vi "SUB_Verify_RandomCode.vi"() -> (1 "Boolean":bool=TRUE)   [LabVIEW 2011]
uses:
  <vilib>/event_ctls.llb/eventvkey.ctl
panel:
  in  "請鍵入如上的驗證碼":string="192.168.1.3\n192.168.1.1\n192.168.1.1"
  out "驗證碼":dbl format="%#_9g"
  # "KT300IP 測點 FAE 使用"
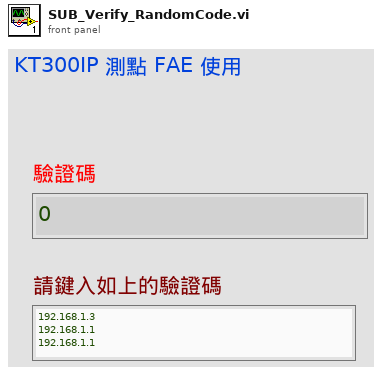
[diagram p1: front panel]
types:
  T1 = typedef "eventvkey.ctl" = enum16{"ASCII", "Enter", "Return", "Shift", "Ctrl", "Alt", "Cmd", "Opt", "Caps", "NumLock", "Clear", "Break", "Up", "Down", "Left", "Right", "Insert", "Delete", "Home", "End", "PageUp", "PageDown", "Escape", "Help", "Pause", "ScrollLock", "F1", "F2", "F3", "F4", "F5", "F6", "F7", "F8", "F9", "F10", "F11", "F12", "F13", "F14", "F15", "F16", "F17", "F18", "F19", "F20", "F21", "F22", "F23", "F24", "Play", "VolumeUp", "VolumeDown", "Mute", "Two Byte Char"}
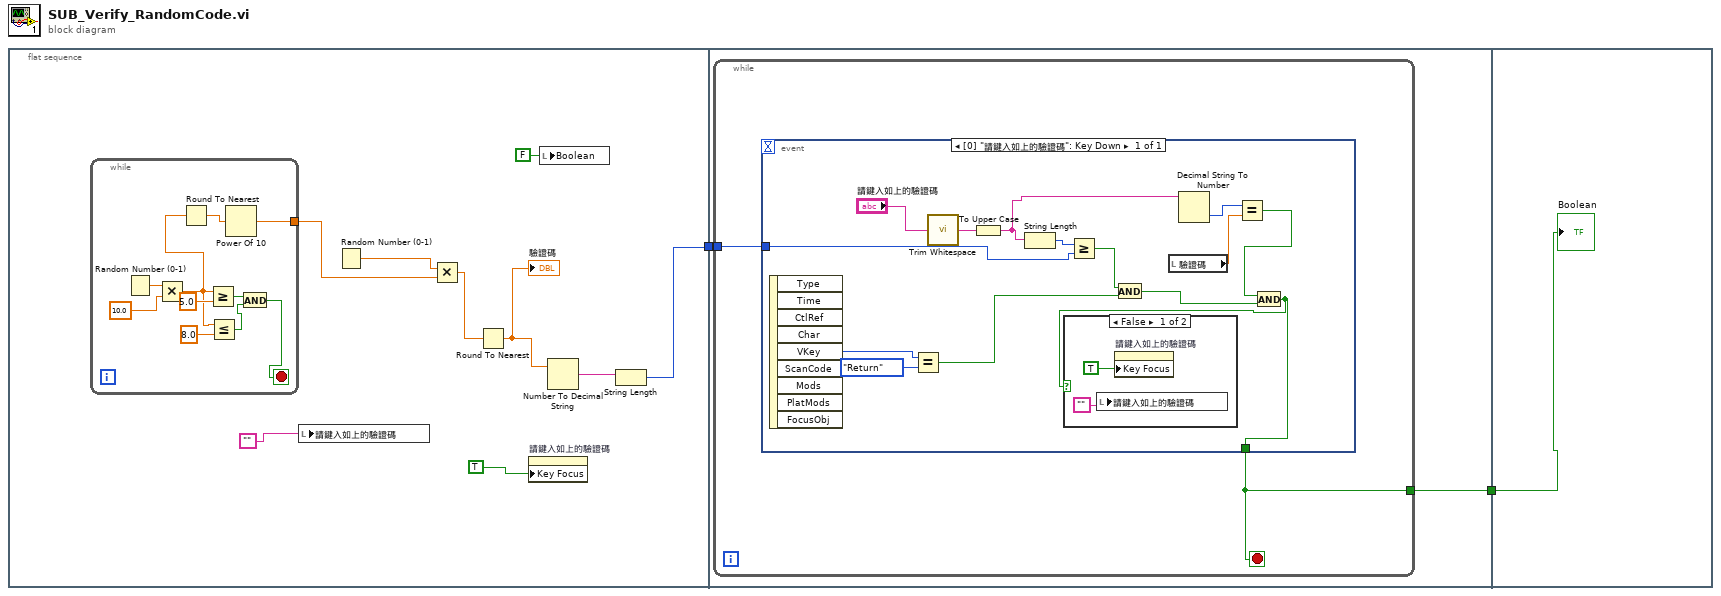
[diagram p0: block diagram]
diagram:
  n1 = flat-sequence {
    tunnel: [w7] -> w2
    tunnel: w2 -> [w23]
    tunnel: [w22] -> w1
    tunnel: w1 -> [w42]
    frame #0 {
      n2 = while {
        tunnel: [w14] -> w3
        stop <- w16 stop-if-true
        n3 = Random Number (0-1)() -> (number: 0 to 1=w21:dbl)
        n4 = Multiply(x=w21, y=10.0) -> (x*y=w13:dbl)
        n5 = Round To Nearest(number=w13) -> (nearest integer value=w12:dbl)
        n6 = Greater Or Equal?(x=w13, y=5.0) -> (x >= y?=w18:bool)
        n7 = Less Or Equal?(x=w13, y=8.0) -> (x <= y?=w17:bool)
        n8 = Power Of 10(x=w12) -> (10^x=w14:dbl)
        n9 = And(x=w18, y=w17) -> (x .and. y?=w16:bool)
      }
      n10 = local write "請鍵入如上的驗證碼"("") -> ()
      n11 = Random Number (0-1)() -> (number: 0 to 1=w11:dbl)
      n12 = Multiply(x=w11, y=w3) -> (x*y=w10:dbl)
      n13 = Round To Nearest(number=w10) -> (nearest integer value=w9:dbl)
      "驗證碼" <- w9
      n14 = property on="請鍵入如上的驗證碼" class="Str"("Key Focus"=TRUE) -> ()  [unwired: 2 in, 2 out]
      n15 = local write "Boolean"(FALSE ("Boolean")) -> ()
      n16 = Number To Decimal String(number=w9) -> (decimal integer string=w8:string)  [unwired: 1 in]
      n17 = String Length(string=w8) -> (length=w7:i32)
    }
    frame #1 {
      n18 = while {
        tunnel: w23 -> [w25]
        tunnel: [w24] -> w22
        stop <- w24 stop-if-true
        n19 = event shown="[0] \"請鍵入如上的驗證碼\": Key Down" {
          selector: _ -> [_]
          dyn-events: _ -> [_]
          timeout: _ -> [_]
          tunnel: w25 -> [w32]
          tunnel: [w26] -> w24
          event "請鍵入如上的驗證碼": Key Down {
            n20 = event-data() -> ("VKey"=w35:T1)  [unwired: 1 in, 8 out]
            n21 = Equal?(x=w35, y=eventvkey."Return") -> (x = y?=w33:bool)
            n22 = call <vilib>:"Trim Whitespace.vi"("string"="請鍵入如上的驗證碼") -> ("trimmed string"=w37:string)  [unwired: 1 in]
            n23 = To Upper Case(1:w37) -> (0:w31:string)
            n24 = String Length(string=w31) -> (length=w39:i32)
            n25 = Greater Or Equal?(x=w39, y=w32) -> (x >= y?=w38:bool)
            n26 = And(x=w38, y=w33) -> (x .and. y?=w27:bool)
            n27 = local read "驗證碼"() -> (w29:dbl)
            n28 = Decimal String To Number(string=w31) -> (number=w30:i32)  [unwired: 2 in, 1 out]
            n29 = Equal?(x=w30, y=w29) -> (x = y?=w28:bool)
            n30 = And(x=w28, y=w27) -> (x .and. y?=w26:bool)
            n31 = case shown="False" w26 {
              frame False {
                n32 = local write "請鍵入如上的驗證碼"("") -> ()
                n33 = property on="請鍵入如上的驗證碼" class="Str"("Key Focus"=TRUE) -> ()  [unwired: 2 in, 2 out]
              }
              frame True {
              }
            }
          }
        }
      }
    }
    frame #2 {
      "Boolean" <- w42
    }
  }
